vi "Test-Intake.vi"() -> ()   [LabVIEW 2023]
doc: "This VI implements the framework and scheduler for your robotics program. It should not be necessary to modify the framework. You are expected to add your code to the VIs called from Robot Main - the ones located in the Team Code folder within the project."
uses:
  <vilib>/Rock Robotics/WPI/DriverStation/WPI_DriverStationRobotMode2.ctl
  <vilib>/Rock Robotics/WPI/Simulation/Protocol/Devices/DriverStation/DS Update Ops.ctl
  <vilib>/Rock Robotics/WPI/ThirdParty/JAS_Junk/TrajLib/VI/BoolCmd_Recv.vi
  <vilib>/Rock Robotics/WPI/ThirdParty/JAS_Junk/TrajLib/VI/BoolCmd_Multiplexor_Array.vi
  Intake/IntakeStateMachine.vi
  <vilib>/Rock Robotics/WPI/ThirdParty/JAS_Junk/TrajLib/VI/BoolCmd_Recv_Internal.vi
  <vilib>/Rock Robotics/WPI/ThirdParty/JAS_Junk/TrajLib/VI/DigSeqLogic_Edge_On.vi
  <vilib>/Rock Robotics/WPI/ThirdParty/JAS_Junk/TrajLib/VI/BoolCmd_ObtainQueue.vi
  Robot Global Data.vi
  Intake/IntakeGlobal.vi
panel:
  out "MotorRPM":dbl format="%9.1f"
  in  "CmdIntake":bool
  in  "CmdSpitOut":bool
  in  "CmdCancel":bool
  out "Robot Mode":T1
  in  "HaveNoteSensor":bool
  out "MotorOutDmd":dbl format="%9.2f"
  in  "error in (no error)":errorcluster
  in  "Finish":bool
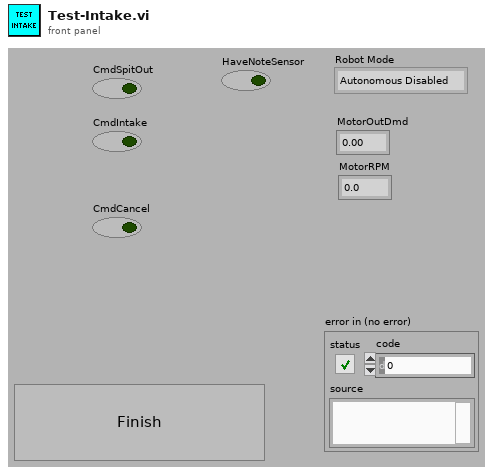
[diagram p1: front panel]
types:
  T1 = typedef "WPI_DriverStationRobotMode2.ctl" = enum16{"Autonomous Disabled", "Autonomous Enabled", "Teleop Disabled", "Teleop Enabled", "Disconnected", "Finish", "Test Disabled", "Test Enabled", "Emergency Stopped"}
  T2 = typedef "WPI_DriverStationMatch Info.ctl" = cluster{"Autonomous Elapsed Seconds":dbl, "TeleOp Elapsed Seconds":dbl, "Disabled Elapsed Seconds":dbl, "Visited Autonomous":bool, "Visited TeleOp":bool, "Visited Disabled":bool, "Autonomous Settings":cluster{"Autonomous Style":enum16{"Iterative", "Independent"}, "VI Refnum":refnum<vi>}}
  T3 = typedef "WPI_DriverStationDerivedRobotMode.ctl" = enum16{"Init", "Execute", "Stop"}
  T4 = typedef "DS Update Ops.ctl" = enum16{"set enabled", "set autonomous", "set test", "set estop", "set fms", "set ds", "set control word", "set match_time", "set station", "set game data", "JSON update", "set name", "get", "transmit initial", "reset"}
  T5 = typedef "NetComm_ControlWord.ctl" = cluster{"Enabled":bool, "Autonomous":bool, "Test":bool, "E-Stop":bool, "FMS Attached":bool, "DS Attached":bool}
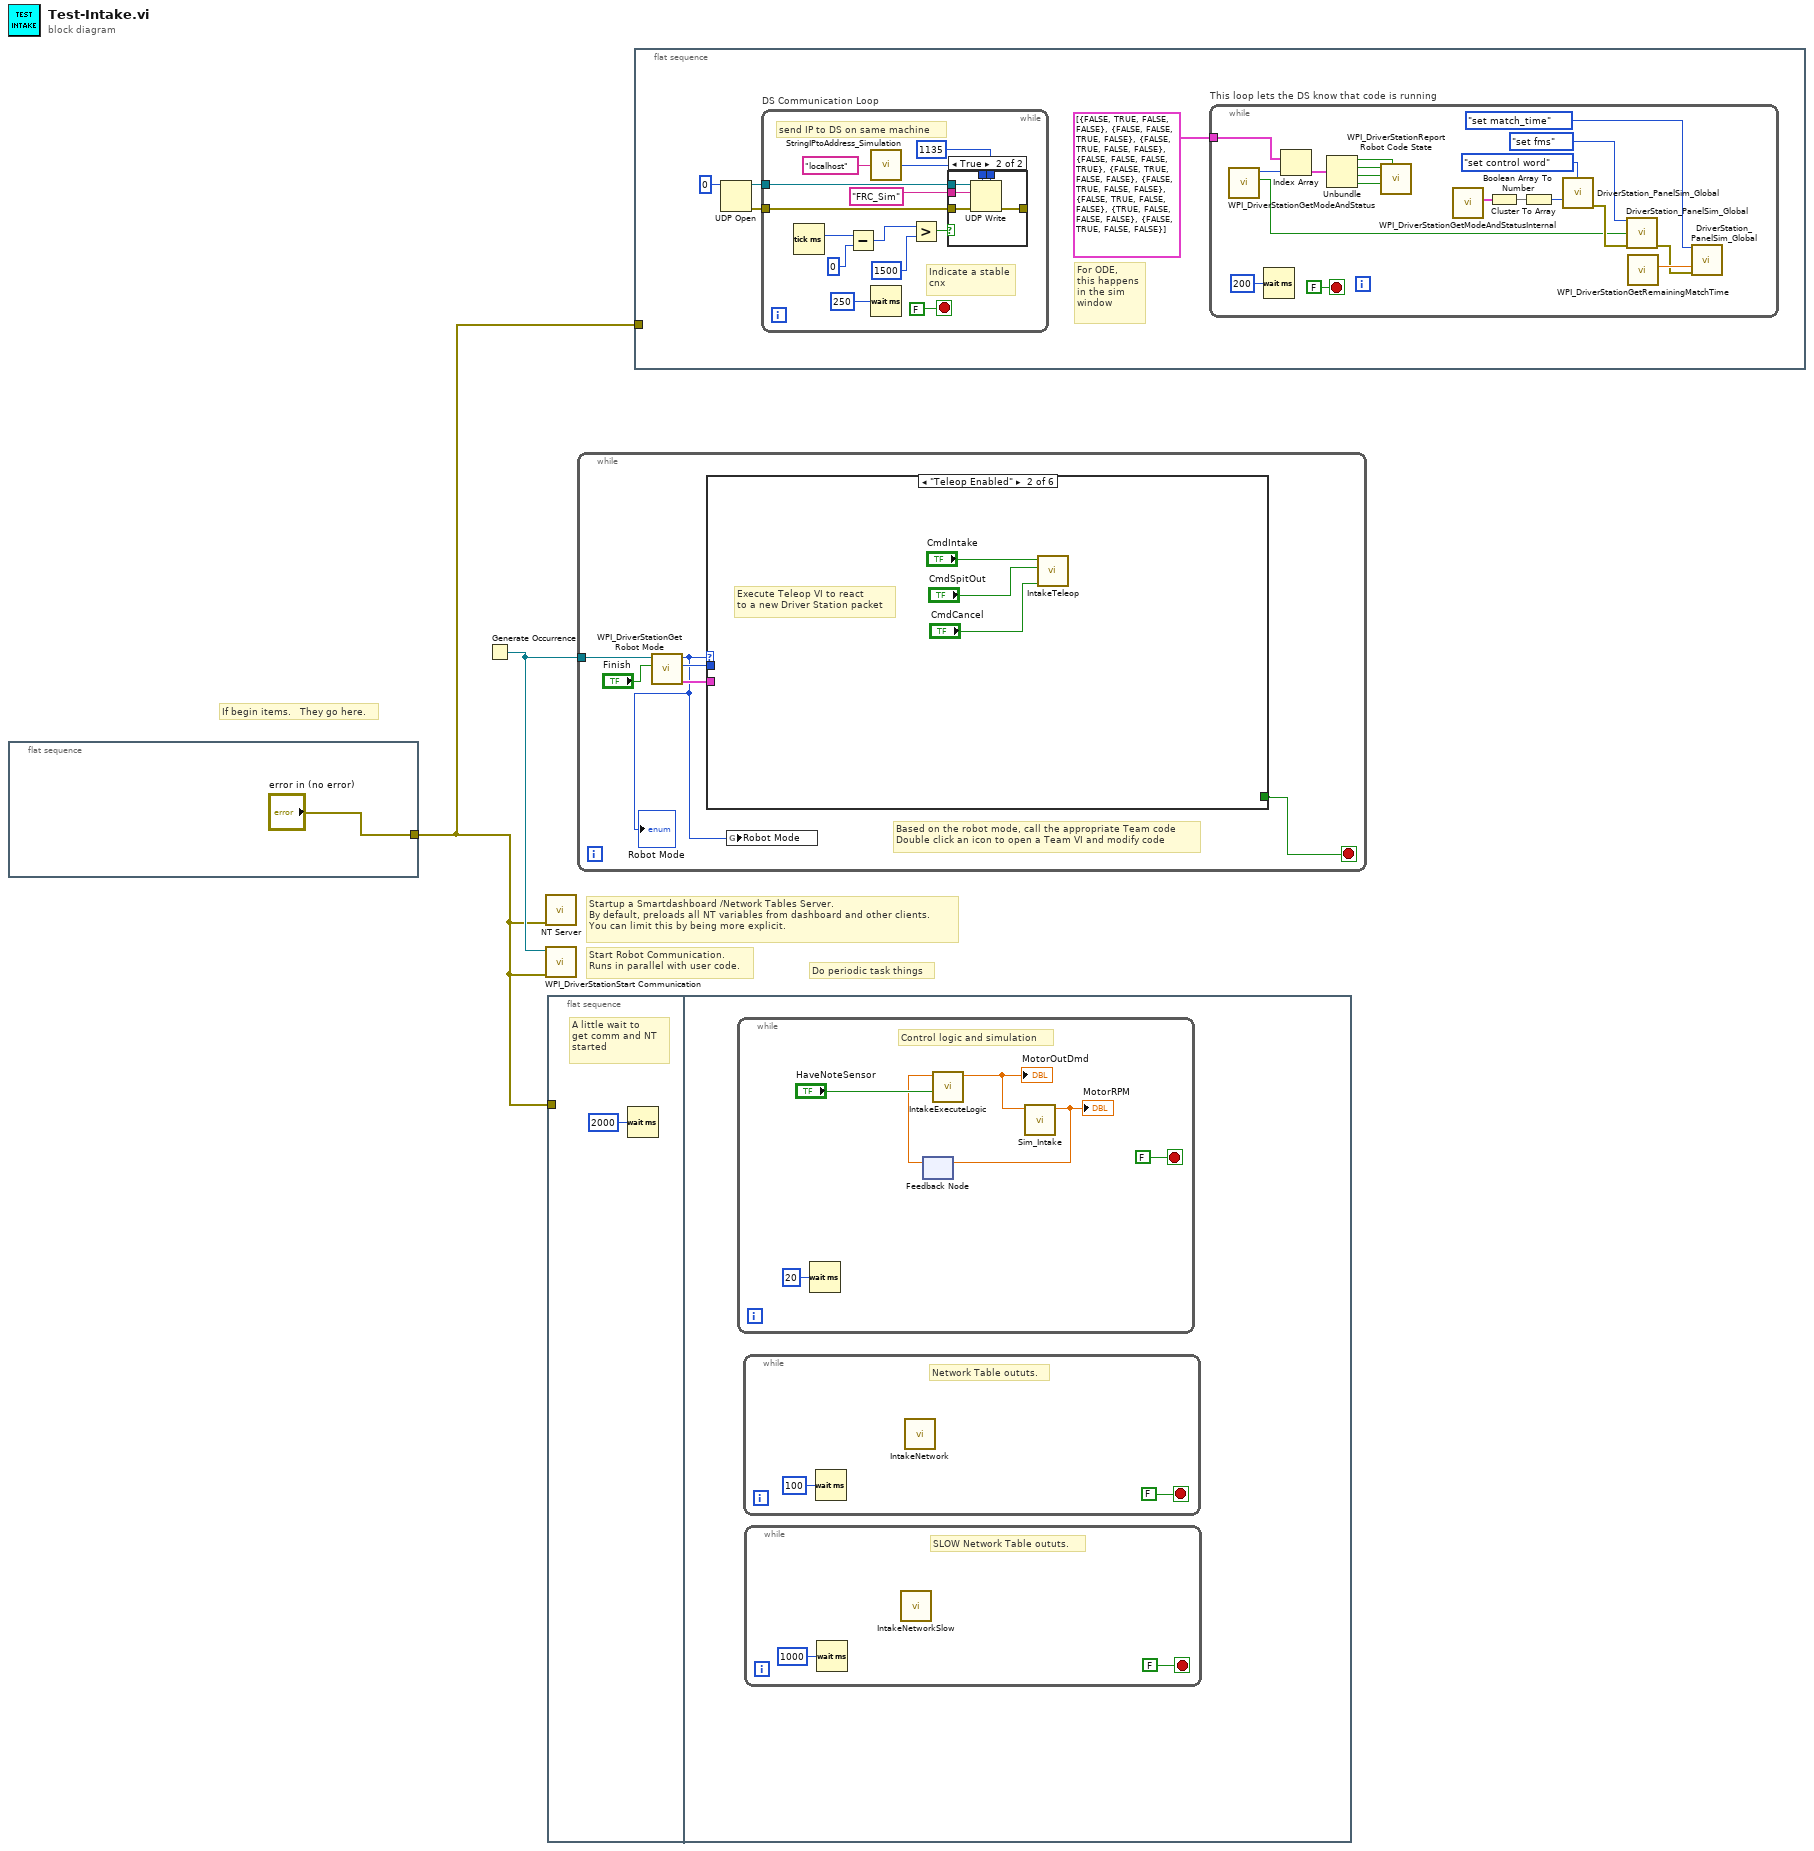
[diagram p0: block diagram]
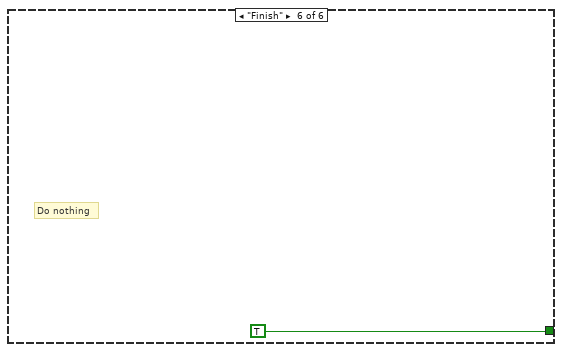
[diagram p6: hidden frame]
diagram:
  # "If begin items.   They go here."
  # "Do periodic task things"
  # "Startup a Smartdashboard /Network Tables Server.\nBy default, preloads all NT variables from dashboard and other clients.\nYou can limit this by being more explicit."
  # "Start Robot Communication.\nRuns in parallel with user code."
  n1 = flat-sequence {
    tunnel: ["error in (no error)"] -> w1
    frame #0 {
    }
  }
  n2 = Generate Occurrence() -> (w2:refnum<k4>)
  n3 = call <vilib>:"NT Server.vi"("error in (no error)"=w1) -> ()  [unwired: 10 in, 1 out]
  n4 = call <vilib>:"WPI_DriverStationStart Communication.vi"("error in (no error)"=w1, "occurrence"=w2) -> ()  [unwired: 1 in, 9 out]
  n5 = flat-sequence {
    tunnel: w1 -> [_]
    frame #0 {
      # "A little wait to\nget comm and NT\nstarted"
      n6 = Wait (ms)(milliseconds to wait=u32 2000) -> ()  [unwired: 1 out]
    }
    frame #1 {
      n7 = while {
        stop <- FALSE stop-if-true
        # "Control logic and simulation"
        n8 = Wait (ms)(milliseconds to wait=u32 20) -> ()  [unwired: 1 out]
        n9 = feedback #1() -> (w10:dbl)  [unwired: 1 in]
        n10 = call "IntakeExecuteLogic.vi"("HaveNoteSensor"="HaveNoteSensor", "Sensor Velocity"=w10) -> ("MotorOutDmd"=w11:dbl)  [unwired: 9 in]
        "MotorOutDmd" <- w11
        n11 = call "Sim_Intake.vi"("Motor Dmd"=w11) -> ("MotorRPM"=w9:dbl)  [unwired: 10 in]
        "MotorRPM" <- w9
        n12 = feedback-in #1(w9) -> ()
      }
      n13 = while {
        stop <- FALSE stop-if-true
        # "Network Table oututs."
        n14 = Wait (ms)(milliseconds to wait=u32 100) -> ()  [unwired: 1 out]
        n15 = call "IntakeNetwork.vi"() -> ()  [unwired: 11 in, 1 out]
      }
      n16 = while {
        stop <- FALSE stop-if-true
        # "SLOW Network Table oututs."
        n17 = Wait (ms)(milliseconds to wait=u32 1000) -> ()  [unwired: 1 out]
        n18 = call "IntakeNetworkSlow.vi"() -> ()  [unwired: 11 in, 1 out]
      }
    }
  }
  n19 = while {
    tunnel: w2 -> [w20]
    stop <- w15 stop-if-true
    # "Based on the robot mode, call the appropriate Team code\nDouble click an icon to open a Team VI and modify code"
    n20 = call <vilib>:"WPI_DriverStationGet Robot Mode.vi"("Finish"="Finish", "DS Occurrence"=w20) -> ("Match Info out"=w17:T2, "Call Context"=w19:T3, "Robot Mode"=w16:T1)  [unwired: 7 out]
    "Robot Mode" <- w16
    n21 = case shown="\"Teleop Enabled\"" w16 {
      tunnel: w19 -> [_ _ _ _ _ _]
      tunnel: w17 -> [_ _ _ _ _ _]
      tunnel: [_ _ _ _ _ TRUE] -> w15
      frame "Autonomous Enabled" {
        # "Do nothing...."
      }
      frame "Teleop Enabled" {
        # "Execute Teleop VI to react\nto a new Driver Station packet"
        n22 = call "IntakeTeleop.vi"("CmdCancel"="CmdCancel", "CmdSpitOut"="CmdSpitOut", "CmdIntake"="CmdIntake") -> ()  [unwired: 9 in]
      }
      frame "Test Disabled", "Test Enabled" {
        # "Do nothing"
      }
      frame "Autonomous Disabled", "Teleop Disabled" {
        # "Do nothing."
      }
      frame "Disconnected", Default {
        # "Driver Station packet didn't arrive.\nPossibly useful for diagnostics"
      }
      frame "Finish" {
        # "Do nothing"
      }
    }
    n23 = global write "Robot Global Data.vi" "Robot Mode"(w16) -> ()
  }
  n24 = flat-sequence {
    tunnel: w1 -> [_]
    frame #0 {
      # "For ODE,\nthis happens\nin the sim\nwindow"
      n25 = UDP Open(11:u16 0 ("port")) -> (port=w28:refnum<k16>, 0:w27:errorcluster)  [unwired: 4 in, 1 out]
      n26 = while "DS Communication Loop" {
        tunnel: w28 -> [w59]
        tunnel: w27 -> [w60]
        stop <- FALSE stop-if-true
        # "Indicate a stable\ncnx"
        # "send IP to DS on same machine"
        n27 = Tick Count (ms)() -> (millisecond timer value=w49:u32)
        n28 = Subtract(x=w49, y=u32 0) -> (x-y=w52:u32)
        n29 = call <vilib>:"StringIPtoAddress_Simulation.vi"("string IP"="localhost" ("DS IP 2")) -> ("address"=w56:u32)  [unwired: 14 in]
        n30 = Wait (ms)(milliseconds to wait=u32 250) -> ()  [unwired: 1 out]
        n31 = Greater?(x=w52, y=u32 1500 ("milliseconds to wait")) -> (0:w50:bool)
        n32 = case shown="True" w50 {
          tunnel: w60 -> [_ w66]
          tunnel: w59 -> [_ w65]
          tunnel: "FRC_Sim" ("data in") -> [_ w64]
          tunnel: w56 -> [_ w63]
          tunnel: [_ w62] -> _
          tunnel: u16 1135 ("port") -> [_ w61]
          frame False {
          }
          frame True {
            n33 = UDP Write(address=w63, port or service name=w61, connection ID=w65, data in=w64, 8:w66) -> (error out=w62:errorcluster)  [unwired: 1 in, 1 out]
          }
        }
      }
      n34 = while "This loop lets the DS know that code is running" {
        tunnel: cluster{bool, bool, bool, bool}[] [{FALSE, TRUE, FALSE, FALSE}, {FALSE, FALSE, TRUE, FALSE}, {FALSE, TRUE, FALSE, FALSE}, {FALSE, FALSE, FALSE, TRUE}, {FALSE, TRUE, FALSE, FALSE}, {FALSE, TRUE, FALSE, FALSE}, {FALSE, TRUE, FALSE, FALSE}, {TRUE, FALSE, FALSE, FALSE}, {FALSE, TRUE, FALSE, FALSE}] -> [w46]
        stop <- FALSE stop-if-true
        n35 = call <vilib>:"WPI_DriverStationGetModeAndStatus.vi"() -> ("FMS Attached"=w29:bool, "Robot Mode"=w40:T1)  [unwired: 10 in]
        n36 = Wait (ms)(milliseconds to wait=u32 200) -> ()  [unwired: 1 out]
        n37 = Index Array(array=w46, index=w40) -> (element=w41:cluster{bool, bool, bool, bool})
        n38 = Unbundle(w41) -> (w47:bool, w39:bool, w44:bool, w43:bool)
        n39 = call <vilib>:"WPI_DriverStationReport Robot Code State.vi"("Test"=w47, "TeleOp"=w43, "Autonomous"=w44, "Disabled"=w39) -> ()  [unwired: 7 in, 1 out]
        n40 = call <vilib>:"WPI_DriverStationGetModeAndStatusInternal.vi"() -> ("Control Word"=w37:T5)  [unwired: 10 in, 1 out]
        n41 = Cluster To Array(cluster=w37) -> (array=w36:bool[])
        n42 = Boolean Array To Number(Boolean array=w36) -> (number=w35:u32)
        n43 = call <vilib>:"DriverStation_PanelSim_Global.vi"("menu"=DS_Update_Ops."set control word", "Numeric Value"=w35) -> ("error out"=w33:errorcluster)  [unwired: 12 in, 1 out]
        n44 = call <vilib>:"DriverStation_PanelSim_Global.vi"("menu"=DS_Update_Ops."set fms", "Value Set"=w29, "error in (no error)"=w33) -> ("error out"=w30:errorcluster)  [unwired: 11 in, 1 out]
        n45 = call <vilib>:"WPI_DriverStationGetRemainingMatchTime.vi"() -> ("Match Time(s)"=w31:sgl)  [unwired: 10 in, 1 out]
        n46 = call <vilib>:"DriverStation_PanelSim_Global.vi"("menu"=DS_Update_Ops."set match_time", "Numeric Value"=w31, "error in (no error)"=w30) -> ()  [unwired: 11 in, 2 out]
      }
    }
  }
